vi "Arduino_address_configure.vi"() -> ()   [LabVIEW 2020]
uses:
  Instrument drivers/Arduino/ctls_and_globals/Arduino tx msg cluster.ctl
panel:
  in  "New address":u8=10
  out "Output":dbl
  out "Status comment":string
  in  "Port":refnum<visa-resource-name>="COM18"
  in  "Current address":u8=255
  # "Use this vi to configure the Arduino's unique address on the RS-485 network.\nRange is 1 - 254. 0 is reserved for master, 255 for first-time config.\nThis value is retained in EEPROM and recalled on power-up."
  # "255 if first time"
  # "1 - 254"
  # "PN 21/01/2014"
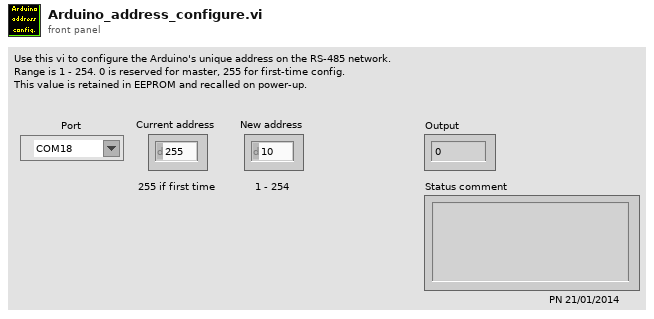
[diagram p1: front panel]
types:
  T1 = typedef "Arduino tx msg cluster.ctl" = cluster{"dest":u8, "A/D/C/I":string, "R/W":string, "chan":u8, "val (float)":sgl}
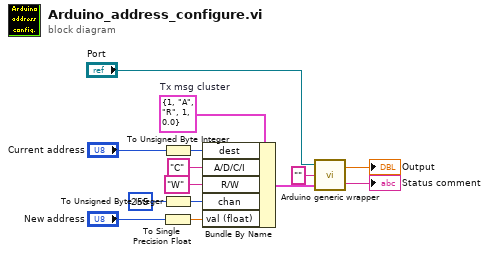
[diagram p0: block diagram]
diagram:
  w10 = T1 {"dest"=1, "A/D/C/I"="A", "R/W"="R", "chan"=1, "val (float)"=0.0}  # Tx msg cluster
  n1 = To Unsigned Byte Integer(number="Current address") -> (unsigned 8bit integer=w6:u8)
  n2 = To Unsigned Byte Integer(number=u8 255) -> (unsigned 8bit integer=w7:u8)
  n3 = To Single Precision Float(number="New address") -> (single precision float=w12:sgl)
  n4 = Bundle By Name(cluster=w10, "dest"=w6, "A/D/C/I"="C" ("A/D"), "R/W"="W", "chan"=w7, "val (float)"=w12) -> (w9:T1)
  n5 = call "Arduino generic wrapper.vi"("Tx msg cluster"=w9, "Channel Name"="", "Port name"="Port") -> ("Scan comment"=→"Status comment":string, "Output"=→"Output":dbl)
